vi "Launcher.vi"() -> ()   [LabVIEW 2020]
uses:
  Digital Acquisition/Digital Acquisition.lvclass
  C:/Program Files (x86)/National Instruments/LabVIEW 2020/vi.lib/ActorFramework/Actor/Actor.lvclass
  <vilib>/ActorFramework/Actor/Actor.lvclass
panel:
  in  "Actor ID":string
  in  "New Digital Acquisition":bool
  in  "New Function Generator":bool
  in  "Close Digital Acquisition":bool
  in  "Close Function Generator":bool
  in  "Digital Acquisition List":i32(listbox)
  in  "Function Generator List":i32(listbox)
  # "Signal Generator and Digital Acquisition"
  # "Developed by Francisco Flores using Actor Framework"
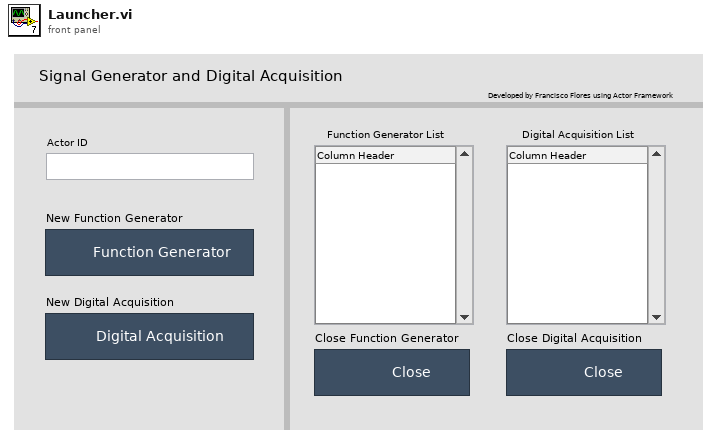
[diagram p1: front panel]
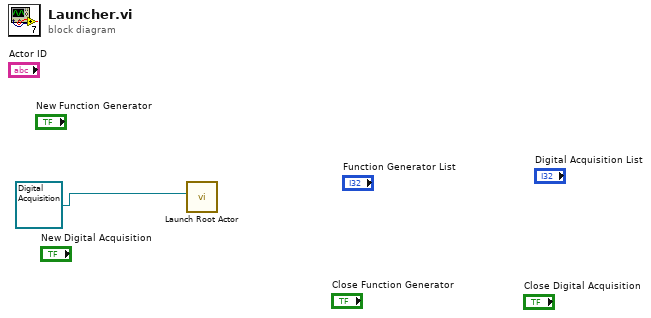
[diagram p0: block diagram]
diagram:
  n1 = call <vilib>:"Launch Root Actor.vi"("Actor"=refnum<class "Digital Acquisition.lvclass"> refnum ("Digital Acquisition.lvlib:Digital Acquisition.lvclass")) -> ()  [unwired: 9 in, 2 out]
